vi "Actor Core.vi"(8 "error in":errorcluster, 11 "DAQ AI in":refnum<class "DAQ AI.lvclass">) -> (0 "error out":errorcluster, 3 "Actor out":refnum<class "Actor.lvclass">)   [LabVIEW 2020, in "DAQ AI.lvlib" / "DAQ AI.lvclass"]
doc: "<p>(<strong>Filename</strong>: <span class=\"dnl\">Actor Framework.lvlib:Actor.lvclass:Actor Core.vi</span>)</p>\n<p>Receives messages to the actor, reacts to them, and initiates any error handling that may shut the actor down.</p>\n<p>Descendant classes may override this VI to append parallel tasks for the actor to complete while it handles messages. Overrides use the <a href=\"nihelplauncher://docs/csh?context=lvcore_glang_udclass\">Call Parent Class Method</a> node.</p>"
uses:
  DAQ AI.lvclass
  <vilib>/ActorFramework/Actor/Actor.lvclass/Actor.ctl
  <vilib>/ActorFramework/Message Enqueuer/Message Enqueuer.lvclass/Message Enqueuer.ctl
  DAQ AI.lvclass/DAQ AI.ctl
  Supervisor/Supervisor Messages/Acquire Waveform Msg/Acquire Waveform Msg.lvclass/Acquire Waveform Msg.ctl
  C:/Program Files (x86)/National Instruments/LabVIEW 2026/vi.lib/ActorFramework/Actor/Actor.lvclass
  C:/Users/taacr/OneDrive/HP/Local/Actor Framework/DAQ AI/DAQ AI/DAQ AI.lvclass
  <vilib>/ActorFramework/Actor/Actor.lvclass
  Supervisor/Supervisor Messages/Acquire Waveform Msg/Acquire Waveform Msg.lvclass
  Supervisor/Supervisor Messages/Over Threshold Msg/Over Threshold Msg.lvclass
panel:
  out "Over Threshold":bool
  out "Waveform Graph":waveform(dbl)[](graph)
  out "DAQmx Analog Channel":tag
  out "Measuring":bool
  out "Period [ms]":i32
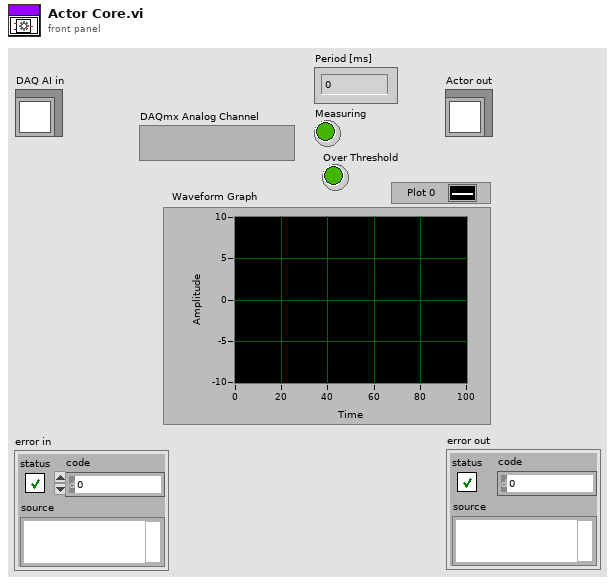
[diagram p1: front panel]
types:
  T1 = typedef "DAQ AI.lvlib/DAQ AI.lvclass/User Events.ctl" = cluster{"Stop Event":refnum<user-event>, "DAQmx Analog Channel Event":refnum<user-event>, "Waveform Graph Event":refnum<user-event>, "Period [ms] Event":refnum<user-event>, "Start/Stop Acquisition Event":refnum<user-event>, "Threshold Event":refnum<user-event>, "Over Threshold Event":refnum<user-event>}
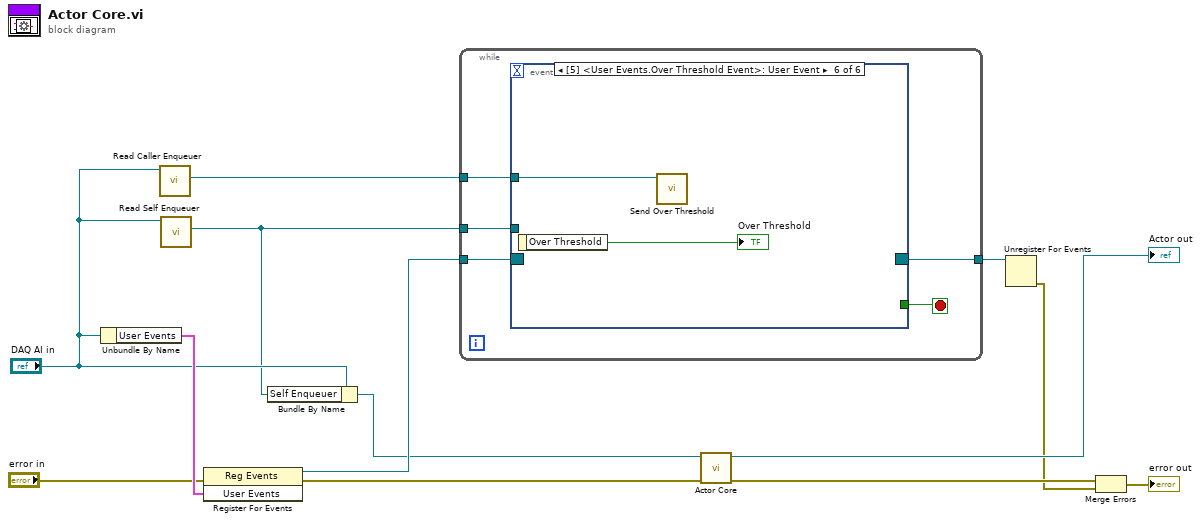
[diagram p0: block diagram]
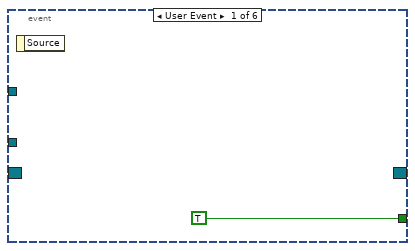
[diagram p2: hidden frame]
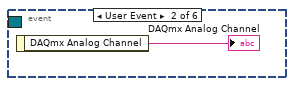
[diagram p3: hidden frame]
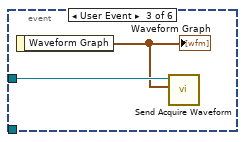
[diagram p4: hidden frame]
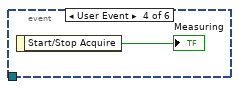
[diagram p5: hidden frame]
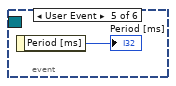
[diagram p6: hidden frame]
diagram:
  n1 = Unbundle By Name("DAQ AI in") -> ("User Events"=w11:T1)
  n2 = call <vilib>:"Read Caller Enqueuer.vi"("Actor"="DAQ AI in") -> ("Caller Enqueuer"=w12:refnum<class "Message Enqueuer.lvclass">)  [unwired: 10 in]
  n3 = call <vilib>:"Read Self Enqueuer.vi"("Actor"="DAQ AI in") -> ("Self Enqueuer"=w2:refnum<class "Message Enqueuer.lvclass">)  [unwired: 10 in]
  n4 = register-events(error in="error in", w11) -> (reference out=w8:refnum<event-registration>, error out=w9:errorcluster)  [unwired: 1 in]
  n5 = Bundle By Name(cluster="DAQ AI in", "Self Enqueuer"=w2) -> (w1:refnum<class "DAQ AI.lvclass">)
  n6 = while {
    tunnel: w12 -> [w18]
    tunnel: w2 -> [w17]
    tunnel: w8 -> [w14]
    tunnel: [w16] -> w7
    stop <- w15 stop-if-true
    n7 = event shown="[5] <User Events.Over Threshold Event>: User Event" {
      selector: w14 -> [_ _ _ _ _ _]
      dyn-events: [_ _ _ _ _ _] -> w16
      timeout: _ -> [_ _ _ _ _ _]
      tunnel: w18 -> [_ _ w22 _ _ w25]
      tunnel: w17 -> [_ _ _ _ _ _]
      tunnel: [TRUE _ _ _ _ _] -> w15
      event User Event {
        n8 = event-data() -> ()  [unwired: 1 in, 1 out]
      }
      event User Event {
        n9 = event-data() -> ("DAQmx Analog Channel"=→"DAQmx Analog Channel":tag)  [unwired: 1 in]
      }
      event User Event {
        n10 = event-data() -> ("Waveform Graph"=w21:waveform(dbl)[])  [unwired: 1 in]
        "Waveform Graph" <- w21
        n11 = call "Send Acquire Waveform.vi"("Waveform Graph"=w21, "Message Enqueuer"=w22) -> ()  [unwired: 8 in, 2 out]
      }
      event User Event {
        n12 = event-data() -> ("Start/Stop Acquire"=→"Measuring":bool)  [unwired: 1 in]
      }
      event User Event {
        n13 = event-data() -> ("Period [ms]"=→"Period [ms]":i32)  [unwired: 1 in]
      }
      event User Event {
        n14 = event-data() -> ("Over Threshold"=→"Over Threshold":bool)  [unwired: 1 in]
        n15 = call "Send Over Threshold.vi"("Message Enqueuer"=w25) -> ()  [unwired: 9 in, 2 out]
      }
    }
  }
  n16 = call-parent "Actor Core.vi"("error in"=w9, "Actor in"=w1) -> ("error out"=w6:errorcluster, "Actor out"=→"Actor out":refnum<class "Actor.lvclass">)  [unwired: 8 in]
  n17 = Unregister For Events(event registration refnum=w7) -> (error out=w5:errorcluster)  [unwired: 1 in]
  n18 = Merge Errors(w6, w5) -> (→"error out":errorcluster)
